vi "ParameterEditor_background_new.vi"(1 "Previous Parameters":T1=[{"Status"="", "Name"="e- block potential (>0 = on)", "Value"=1.0, "Changed"=FALSE}, {"Status"="", "Name"="e- filament bias (V)", "Value"=6.3, "Changed"=FALSE}, {"Status"="", "Name"="e- current (A) [0.3 A limit]", "Value"=0.0, "Changed"=FALSE}, {"Status"="", "Name"="e- ramp time (s)", "Value"=40.0, "Changed"=FALSE}, {"Status"="", "Name"="e- source ON (1 or 0)", "Value"=1.0, "Changed"=FALSE}, {"Status"="", "Name"="", "Value"=0.0, "Changed"=FALSE}, {"Status"="", "Name"="e+ accumulation time (s)", "Value"=0.0, "Changed"=FALSE}, {"Status"="", "Name"="e+ escape energy (eV)", "Value"=0.0, "Changed"=FALSE}, {"Status"="", "Name"="", "Value"=0.0, "Changed"=FALSE}, {"Status"="", "Name"="HV pulse enable (1 or 0)", "Value"=0.0, "Changed"=FALSE}, {"Status"="", "Name"="HV pulse channel", "Value"=0.0, "Changed"=FALSE}, {"Status"="", "Name"="HV pulse voltage", "Value"=0.0, "Changed"=FALSE}, {"Status"="", "Name"="", "Value"=0.0, "Changed"=FALSE}, {"Status"="", "Name"="Tanaka enable (1 or 0)", "Value"=0.0, "Changed"=FALSE}, {"Status"="", "Name"="", "Value"=0.0, "Changed"=FALSE}, {"Status"="", "Name"="MCP front bias (divided by 400 V)", "Value"=0.0, "Changed"=FALSE}, {"Status"="", "Name"="MCP back bias (divided by 400 V)", "Value"=0.0, "Changed"=FALSE}, {"Status"="", "Name"="Phosphor bias (divided by 400 V)", "Value"=0.0, "Changed"=FALSE}, {"Status"="", "Name"="", "Value"=0.0, "Changed"=FALSE}, {"Status"="", "Name"="US RW ON (1 or 0)", "Value"=0.0, "Changed"=FALSE}, {"Status"="", "Name"="US RW frequency (Hz)", "Value"=300000.0, "Changed"=FALSE}, {"Status"="", "Name"="US RW amplitude (V)", "Value"=1.0, "Changed"=FALSE}, {"Status"="", "Name"="US RW phase 1 (degrees)", "Value"=0.0, "Changed"=FALSE}, {"Status"="", "Name"="US RW phase 2 (degrees)", "Value"=-90.0, "Changed"=FALSE}, {"Status"="", "Name"="US RW sweep time (s)", "Value"=20.0, "Changed"=FALSE}, {"Status"="", "Name"="", "Value"=0.0, "Changed"=FALSE}, {"Status"="", "Name"="DS RW ON (1 or 0)", "Value"=0.0, "Changed"=FALSE}, {"Status"="", "Name"="DS RW frequency (Hz)", "Value"=0.0, "Changed"=FALSE}, {"Status"="", "Name"="DS RW amplitude (V)", "Value"=0.0, "Changed"=FALSE}, {"Status"="", "Name"="DS RW phase 1 (degrees)", "Value"=0.0, "Changed"=FALSE}, {"Status"="", "Name"="DS RW phase 2 (degrees)", "Value"=0.0, "Changed"=FALSE}, {"Status"="", "Name"="DS RW sweep time (s)", "Value"=0.0, "Changed"=FALSE}, {"Status"="", "Name"="", "Value"=0.0, "Changed"=FALSE}, {"Status"="", "Name"="dg645 AB delay (ns)", "Value"=0.0, "Changed"=FALSE}, {"Status"="", "Name"="dg645 AB width (ns)", "Value"=0.0, "Changed"=FALSE}, {"Status"="", "Name"="dg645 CD delay (ns)", "Value"=0.0, "Changed"=FALSE}, {"Status"="", "Name"="dg645 CD width (ns)", "Value"=0.0, "Changed"=FALSE}, {"Status"="", "Name"="dg645 EF delay (ns)", "Value"=0.0, "Changed"=FALSE}, {"Status"="", "Name"="dg645 EF width (ns)", "Value"=0.0, "Changed"=FALSE}, {"Status"="", "Name"="dg645 GH delay (ns)", "Value"=0.0, "Changed"=FALSE}, {"Status"="", "Name"="dg645 GH width (ns)", "Value"=0.0, "Changed"=FALSE}] {"Value" format="%_6p"}, 2 "New Parameters":T1=[{"Status"="", "Name"="e- block potential (>0 = on)", "Value"=0.0, "Changed"=TRUE}, {"Status"="", "Name"="e- filament bias (V)", "Value"=0.1, "Changed"=TRUE}, {"Status"="", "Name"="e- current (A) [0.3 A limit]", "Value"=0.0, "Changed"=FALSE}, {"Status"="", "Name"="e- ramp time (s)", "Value"=40.0, "Changed"=FALSE}, {"Status"="", "Name"="e- source ON (1 or 0)", "Value"=0.0, "Changed"=TRUE}, {"Status"="", "Name"="", "Value"=0.0, "Changed"=FALSE}, {"Status"="", "Name"="e+ accumulation time (s)", "Value"=0.0, "Changed"=FALSE}, {"Status"="", "Name"="e+ escape energy (eV)", "Value"=0.0, "Changed"=FALSE}, {"Status"="", "Name"="", "Value"=0.0, "Changed"=FALSE}, {"Status"="", "Name"="HV pulse enable (1 or 0)", "Value"=0.0, "Changed"=FALSE}, {"Status"="", "Name"="HV pulse channel", "Value"=0.0, "Changed"=FALSE}, {"Status"="", "Name"="HV pulse voltage", "Value"=0.0, "Changed"=FALSE}, {"Status"="", "Name"="", "Value"=0.0, "Changed"=FALSE}, {"Status"="", "Name"="Tanaka enable (1 or 0)", "Value"=0.0, "Changed"=FALSE}, {"Status"="", "Name"="", "Value"=0.0, "Changed"=FALSE}, {"Status"="", "Name"="MCP front bias (divided by 400 V)", "Value"=0.0, "Changed"=FALSE}, {"Status"="", "Name"="MCP back bias (divided by 400 V)", "Value"=0.0, "Changed"=FALSE}, {"Status"="", "Name"="Phosphor bias (divided by 400 V)", "Value"=0.0, "Changed"=FALSE}, {"Status"="", "Name"="", "Value"=0.0, "Changed"=FALSE}, {"Status"="", "Name"="US RW ON (1 or 0)", "Value"=0.0, "Changed"=FALSE}, {"Status"="", "Name"="US RW frequency (Hz)", "Value"=300000.0, "Changed"=FALSE}, {"Status"="", "Name"="US RW amplitude (V)", "Value"=1.0, "Changed"=FALSE}, {"Status"="", "Name"="US RW phase 1 (degrees)", "Value"=0.0, "Changed"=FALSE}, {"Status"="", "Name"="US RW phase 2 (degrees)", "Value"=-90.0, "Changed"=FALSE}, {"Status"="", "Name"="US RW sweep time (s)", "Value"=20.0, "Changed"=FALSE}, {"Status"="", "Name"="", "Value"=0.0, "Changed"=FALSE}, {"Status"="", "Name"="DS RW ON (1 or 0)", "Value"=0.0, "Changed"=FALSE}, {"Status"="", "Name"="DS RW frequency (Hz)", "Value"=0.0, "Changed"=FALSE}, {"Status"="", "Name"="DS RW amplitude (V)", "Value"=0.0, "Changed"=FALSE}, {"Status"="", "Name"="DS RW phase 1 (degrees)", "Value"=0.0, "Changed"=FALSE}, {"Status"="", "Name"="DS RW phase 2 (degrees)", "Value"=0.0, "Changed"=FALSE}, {"Status"="", "Name"="DS RW sweep time (s)", "Value"=0.0, "Changed"=FALSE}, {"Status"="", "Name"="", "Value"=0.0, "Changed"=FALSE}, {"Status"="", "Name"="dg645 AB delay (ns)", "Value"=0.0, "Changed"=FALSE}, {"Status"="", "Name"="dg645 AB width (ns)", "Value"=0.0, "Changed"=FALSE}, {"Status"="", "Name"="dg645 CD delay (ns)", "Value"=0.0, "Changed"=FALSE}, {"Status"="", "Name"="dg645 CD width (ns)", "Value"=0.0, "Changed"=FALSE}, {"Status"="", "Name"="dg645 EF delay (ns)", "Value"=0.0, "Changed"=FALSE}, {"Status"="", "Name"="dg645 EF width (ns)", "Value"=0.0, "Changed"=FALSE}, {"Status"="", "Name"="dg645 GH delay (ns)", "Value"=0.0, "Changed"=FALSE}, {"Status"="", "Name"="dg645 GH width (ns)", "Value"=0.0, "Changed"=FALSE}] {"Value" format="%_6p"}) -> (0 "Output parameters":T1=[{"Status"="", "Name"="e- block potential (>0 = on)", "Value"=0.0, "Changed"=TRUE}, {"Status"="", "Name"="e- filament bias (V)", "Value"=0.1, "Changed"=TRUE}, {"Status"="", "Name"="e- current (A) [0.3 A limit]", "Value"=0.0, "Changed"=FALSE}, {"Status"="", "Name"="e- ramp time (s)", "Value"=40.0, "Changed"=FALSE}, {"Status"="", "Name"="e- source ON (1 or 0)", "Value"=0.0, "Changed"=TRUE}, {"Status"="", "Name"="", "Value"=0.0, "Changed"=FALSE}, {"Status"="", "Name"="e+ accumulation time (s)", "Value"=0.0, "Changed"=FALSE}, {"Status"="", "Name"="e+ escape energy (eV)", "Value"=0.0, "Changed"=FALSE}, {"Status"="", "Name"="", "Value"=0.0, "Changed"=FALSE}, {"Status"="", "Name"="HV pulse enable (1 or 0)", "Value"=0.0, "Changed"=FALSE}, {"Status"="", "Name"="HV pulse channel", "Value"=0.0, "Changed"=FALSE}, {"Status"="", "Name"="HV pulse voltage", "Value"=0.0, "Changed"=FALSE}, {"Status"="", "Name"="", "Value"=0.0, "Changed"=FALSE}, {"Status"="", "Name"="Tanaka enable (1 or 0)", "Value"=0.0, "Changed"=FALSE}, {"Status"="", "Name"="", "Value"=0.0, "Changed"=FALSE}, {"Status"="", "Name"="MCP front bias (divided by 400 V)", "Value"=0.0, "Changed"=FALSE}, {"Status"="", "Name"="MCP back bias (divided by 400 V)", "Value"=0.0, "Changed"=FALSE}, {"Status"="", "Name"="Phosphor bias (divided by 400 V)", "Value"=0.0, "Changed"=FALSE}, {"Status"="", "Name"="", "Value"=0.0, "Changed"=FALSE}, {"Status"="", "Name"="US RW ON (1 or 0)", "Value"=0.0, "Changed"=FALSE}, {"Status"="", "Name"="US RW frequency (Hz)", "Value"=300000.0, "Changed"=FALSE}, {"Status"="", "Name"="US RW amplitude (V)", "Value"=1.0, "Changed"=FALSE}, {"Status"="", "Name"="US RW phase 1 (degrees)", "Value"=0.0, "Changed"=FALSE}, {"Status"="", "Name"="US RW phase 2 (degrees)", "Value"=-90.0, "Changed"=FALSE}, {"Status"="", "Name"="US RW sweep time (s)", "Value"=20.0, "Changed"=FALSE}, {"Status"="", "Name"="", "Value"=0.0, "Changed"=FALSE}, {"Status"="", "Name"="DS RW ON (1 or 0)", "Value"=0.0, "Changed"=FALSE}, {"Status"="", "Name"="DS RW frequency (Hz)", "Value"=0.0, "Changed"=FALSE}, {"Status"="", "Name"="DS RW amplitude (V)", "Value"=0.0, "Changed"=FALSE}, {"Status"="", "Name"="DS RW phase 1 (degrees)", "Value"=0.0, "Changed"=FALSE}, {"Status"="", "Name"="DS RW phase 2 (degrees)", "Value"=0.0, "Changed"=FALSE}, {"Status"="", "Name"="DS RW sweep time (s)", "Value"=0.0, "Changed"=FALSE}, {"Status"="", "Name"="", "Value"=0.0, "Changed"=FALSE}, {"Status"="", "Name"="dg645 AB delay (ns)", "Value"=0.0, "Changed"=FALSE}, {"Status"="", "Name"="dg645 AB width (ns)", "Value"=0.0, "Changed"=FALSE}, {"Status"="", "Name"="dg645 CD delay (ns)", "Value"=0.0, "Changed"=FALSE}, {"Status"="", "Name"="dg645 CD width (ns)", "Value"=0.0, "Changed"=FALSE}, {"Status"="", "Name"="dg645 EF delay (ns)", "Value"=0.0, "Changed"=FALSE}, {"Status"="", "Name"="dg645 EF width (ns)", "Value"=0.0, "Changed"=FALSE}, {"Status"="", "Name"="dg645 GH delay (ns)", "Value"=0.0, "Changed"=FALSE}, {"Status"="", "Name"="dg645 GH width (ns)", "Value"=0.0, "Changed"=FALSE}] {"Value" format="%_6p"})   [LabVIEW 2018]
uses:
  Parameters.ctl
panel:
  in  "Parameter History":enum32{"New", "Previous", "Output"}(tab)
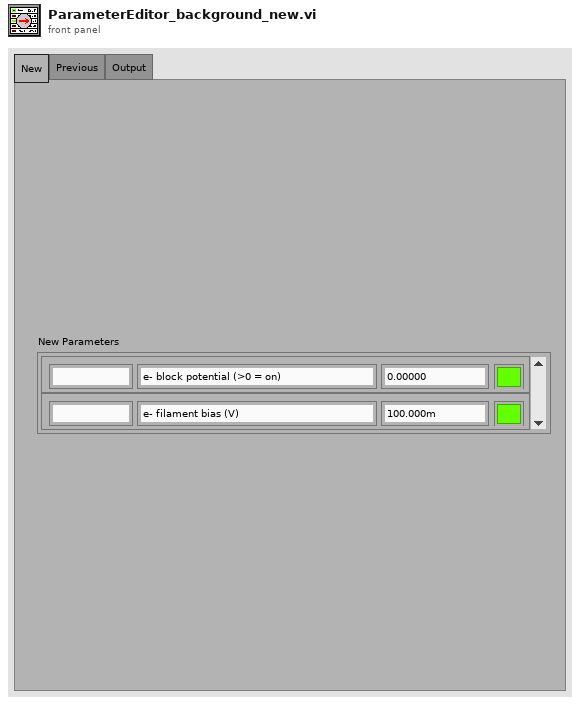
[diagram p1: front panel]
types:
  T1 = typedef "Parameters.ctl" = cluster{"Status":string, "Name":string, "Value":dbl, "Changed":bool}[]
  T2 = cluster{"Status":string, "Name":string, "Value":dbl, "Changed":bool}
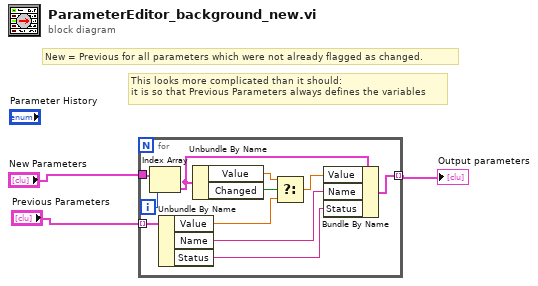
[diagram p0: block diagram]
diagram:
  # "This looks more complicated than it should:\nit is so that Previous Parameters always defines the variables"
  # "New = Previous for all parameters which were not already flagged as changed."
  n1 = for {
    tunnel: "New Parameters" -> [w8]
    tunnel: "Previous Parameters" -> [w14] mode=indexing
    tunnel: [w13] -> w1 mode=indexing
    i -> [w7]
    n2 = Index Array(array=w8, index=w7) -> (element=w6:T2)
    n3 = Unbundle By Name(w14) -> ("Value"=w10:dbl, "Name"=w5:string, "Status"=w4:string)
    n4 = Unbundle By Name(w6) -> ("Value"=w12:dbl, "Changed"=w11:bool)
    n5 = Select(t=w12, s=w11, f=w10) -> (s? t:f=w9:dbl)
    n6 = Bundle By Name(cluster=w6, "Value"=w9, "Name"=w5, "Status"=w4) -> (w13:T2)
  }
  "Output parameters" <- w1
